vi "performSingleRefCalibration.vi"(7 "io_timeout":u16, 8 "error in":errorcluster, 9 "vhv_init_byte":u8, 10 "Slave Address (7-bit)":u8, 11 "I2C Ref In":T1) -> (0 "error out":errorcluster, 2 "status":bool, 3 "I2C Ref Out":T1)   [LabVIEW 2018]
uses:
  <vilib>/myRIO/Instrument Drivers/Onboard IO/I2C/typedefs/I2C Reference.ctl
  <vilib>/myRIO/Common/Instrument Driver Framework/Utilities/typedefs/myRIO Generic Hardware Reference.ctl
  <vilib>/myRIO/Common/Instrument Driver Framework/Utilities/typedefs/Hardware Version Enum.ctl
  <vilib>/myRIO/Common/Instrument Driver Framework/Utilities/typedefs/myRIO v1.0 Reference.ctl
  <vilib>/myRIO/Common/Instrument Driver Framework/Utilities/typedefs/Generic FPGA Reference.ctl
  <vilib>/myRIO/Common/Instrument Driver Framework/myRIO v1.0/I2C/typedefs/I2C Channels Enum.ctl
  <vilib>/myRIO/Instrument Drivers/Onboard IO/I2C/typedefs/I2C Configuration.ctl
  <vilib>/myRIO/Instrument Drivers/Onboard IO/I2C/typedefs/I2C Transfer Rate.ctl
  <vilib>/Utility/error.llb/Error Cluster From Error Code.vi
  <vilib>/myRIO/Common/Instrument Driver Framework/myRIO v1.0/I2C/vis/myRIO v1.0 Write I2C.vi
  <vilib>/myRIO/Common/Instrument Driver Framework/myRIO v1.0/I2C/vis/myRIO v1.0 Read I2C.vi
  <vilib>/myRIO/Instrument Drivers/Onboard IO/I2C/I2C.lvlib
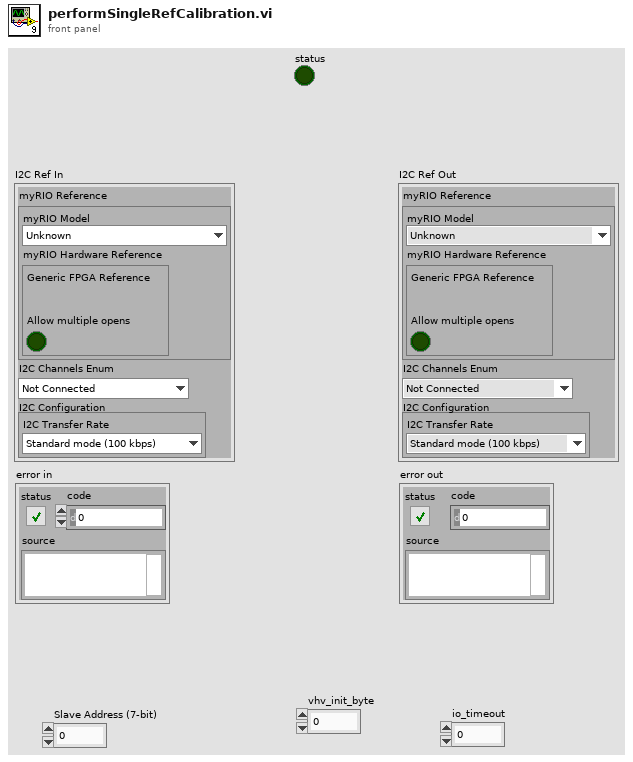
[diagram p1: front panel]
types:
  T1 = typedef "I2C.lvlib/I2C Reference.ctl" = cluster{"myRIO Reference":T2, "I2C Channels Enum":T6, "I2C Configuration":T7}
  T2 = typedef "myRIO Generic Hardware Reference.ctl" = cluster{"myRIO Model":T3, "myRIO Hardware Reference":T4}
  T3 = typedef "Hardware Version Enum.ctl" = enum16{"Unknown", "myRIO-1900", "myRIO-1950", "roboRIO", "NI ELVIS RIO CM", "ELVIS III"}
  T4 = typedef "myRIO v1.0 Reference.ctl" = cluster{"Generic FPGA Reference":T5, "Allow multiple opens":bool}
  T5 = typedef "Generic FPGA Reference.ctl" = refnum<k20>
  T6 = typedef "I2C Channels Enum.ctl" = enum16{"Not Connected", "A/I2C", "B/I2C", "I2C/I2C"}
  T7 = typedef "I2C.lvlib/I2C Configuration.ctl" = cluster{"I2C Transfer Rate":T8}
  T8 = typedef "I2C.lvlib/I2C Transfer Rate.ctl" = enum16{"Standard mode (100 kbps)", "Fast mode (400 kbps)"}
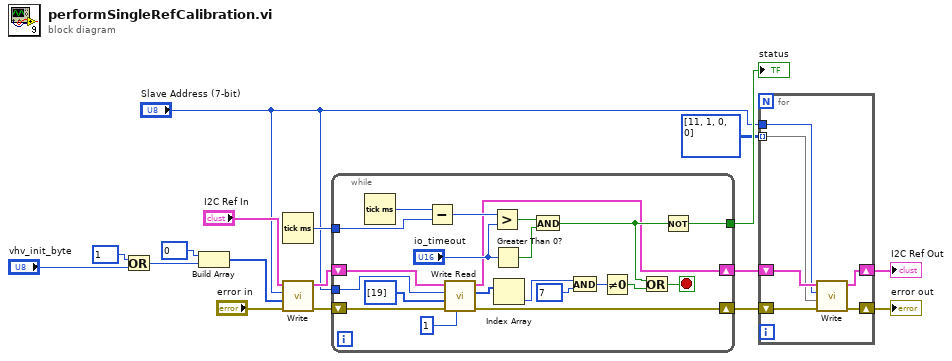
[diagram p0: block diagram]
diagram:
  n1 = Or(x=u8 1, y="vhv_init_byte") -> (x .or. y?=w15:u8)
  n2 = Build Array(u8 0, w15) -> (w11:u8[])
  n3 = Tick Count (ms)() -> (millisecond timer value=w13:u32)
  n4 = call <vilib>:"Write.vi"("error in (no error)"="error in", "Bytes to Write"=w11, "Slave Address (7-bit)"="Slave Address (7-bit)", "I2C Ref In"="I2C Ref In") -> ("error out"=w8:errorcluster, "I2C Ref Out"=w9:T1)  [unwired: 6 in]
  n5 = while {
    tunnel: w13 -> [w28]
    tunnel: "Slave Address (7-bit)" -> [w36]
    tunnel: [w18] -> w7
    shift-right: [w20] -> w5
    shift-left: w9 -> [w38]
    shift-right: [w19] -> w4
    shift-left: w8 -> [w37]
    stop <- w22 stop-if-true
    n6 = Tick Count (ms)() -> (millisecond timer value=w29:u32)
    n7 = Subtract(x=w29, y=w28) -> (x-y=w27:u32)
    n8 = call <vilib>:"Write Read.vi"("Byte Count"=u32 1, "error in (no error)"=w37, "Bytes to Write"=u8[] [19], "Slave Address (7-bit)"=w36, "I2C Ref In"=w38) -> ("error out"=w19:errorcluster, "Bytes Read"=w33:u8[], "I2C Ref Out"=w20:T1)  [unwired: 3 in]
    n9 = Greater?(x=w27, y="io_timeout") -> (0:w24:bool)
    n10 = Greater Than 0?(x="io_timeout") -> (x > 0?=w25:bool)
    n11 = Index Array(array=w33) -> (element=w32:u8)  [unwired: 1 in]
    n12 = And(x=w24, y=w25) -> (x .and. y?=w21:bool)
    n13 = And(x=w32, y=u8 7) -> (x .and. y?=w30:u8)
    n14 = Not Equal To 0?(x=w30) -> (x != 0?=w23:bool)
    n15 = Or(x=w21, y=w23) -> (x .or. y?=w22:bool)
    n16 = Not(x=w21) -> (.not. x?=w18:bool)
  }
  "status" <- w7
  n17 = for {
    tunnel: u8[][] [[11, 1], [0, 0]] -> [w41] mode=indexing
    shift-right: [w40] -> w2
    shift-left: w5 -> [w44]
    shift-right: [w39] -> w1
    shift-left: w4 -> [w43]
    tunnel: "Slave Address (7-bit)" -> [w42]
    n18 = call <vilib>:"Write.vi"("error in (no error)"=w43, "Bytes to Write"=w41, "Slave Address (7-bit)"=w42, "I2C Ref In"=w44) -> ("error out"=w39:errorcluster, "I2C Ref Out"=w40:T1)  [unwired: 6 in]
  }
  "I2C Ref Out" <- w2
  "error out" <- w1
